vi "SP_OEE_2_test.vi"() -> ()   [LabVIEW 2017] (continued)
                      tunnel: w11433 -> [w11683]
                      tunnel: w11432 -> [w11682]
                      tunnel: w11431 -> [w11677]
                      tunnel: w11430 -> [w11679]
                      tunnel: w11429 -> [w11681]
                      tunnel: w11428 -> [w11680]
                      tunnel: w11427 -> [w11674]
                      tunnel: w11426 -> [w11675]
                      tunnel: [w11688] -> w11422
                      tunnel: [w11687] -> w11421
                      tunnel: [w11686] -> w11420
                      tunnel: [w11685] -> w11419
                      tunnel: [w11684] -> w11418
                      tunnel: [w11683] -> w11417
                      tunnel: [w11682] -> w11416
                      tunnel: [w11681] -> w11415
                      tunnel: [w11680] -> w11414
                      tunnel: [w11678] -> w11413
                      tunnel: [w11676] -> w11412
                      tunnel: [w11672] -> w11411
                      tunnel: [w11670] -> w11410
                      tunnel: w11425 -> [w11671]
                      tunnel: w11424 -> [w11667]
                      tunnel: [w11666] -> w11409
                      tunnel: w11423 -> [w11666]
                      tunnel: w11422 -> [w11727]
                      tunnel: w11421 -> [w11720]
                      tunnel: w11420 -> [w11711]
                      tunnel: w11419 -> [w11719]
                      tunnel: w11418 -> [w11709]
                      tunnel: w11417 -> [w11718]
                      tunnel: w11416 -> [w11707]
                      tunnel: w11415 -> [w11717]
                      tunnel: w11414 -> [w11705]
                      tunnel: w11413 -> [w11741]
                      tunnel: w11412 -> [w11740]
                      tunnel: w11411 -> [w11716]
                      tunnel: w11410 -> [w11703]
                      tunnel: [w11741] -> w11408
                      tunnel: [w11740] -> w11407
                      tunnel: [w11734] -> w11406
                      tunnel: [w11727] -> w11405
                      tunnel: [w11726] -> w11404
                      tunnel: [w11725] -> w11403
                      tunnel: [w11724] -> w11402
                      tunnel: [w11723] -> w11401
                      tunnel: [w11722] -> w11400
                      tunnel: [w11721] -> w11399
                      tunnel: [w11720] -> w11398
                      tunnel: [w11719] -> w11397
                      tunnel: [w11718] -> w11396
                      tunnel: [w11717] -> w11395
                      tunnel: [w11716] -> w11394
                      tunnel: [w11701] -> w11393
                      tunnel: w11409 -> [w11701]
                      tunnel: [w11754] -> _
                      tunnel: [w11748] -> _
                      tunnel: w11408 -> [w11749]
                      tunnel: w11407 -> [w11754]
                      tunnel: w11406 -> [w11743]
                      tunnel: w11405 -> [w11752]
                      tunnel: w11404 -> [w11750]
                      tunnel: w11403 -> [_]
                      tunnel: w11402 -> [_]
                      tunnel: w11401 -> [_]
                      tunnel: w11400 -> [_]
                      tunnel: w11399 -> [w11744]
                      tunnel: w11398 -> [w11751]
                      tunnel: w11397 -> [_]
                      tunnel: w11396 -> [_]
                      tunnel: w11395 -> [_]
                      tunnel: w11394 -> [_]
                      tunnel: w11393 -> [w11747]
                      frame #0 {
                        w11497 = "%Y-%m-%d" ("time format string (%c)")
                        n2093 = Decimal String To Number(string=w11483) -> (number=w11484:i32)  [unwired: 2 in, 1 out]
                        n2094 = property on="Table" class="Tbl (strict)"("Visible"=TRUE) -> ()  [unwired: 2 in, 2 out]
                        n2095 = Format Date/Time String(time format string (%c)=w11497, seconds (now)=w11489) -> (date/time string=w11498:string)  [unwired: 1 in]
                        n2096 = Format Date/Time String(time format string (%c)=w11497, seconds (now)=w11488) -> (date/time string=w11496:string)  [unwired: 1 in]
                        n2097 = Format Into String(format string="Where BREAKDOWN_DATE between '%s' and '%s' and  SHIFT_ID = '%d'  ", w11498, w11496, w11484) -> (resulting string=w11495:string)  [unwired: 2 in, 1 out]
                        n2098 = call <vilib>:"DB Tools Select Data.vi"("condition"=w11495, "error in (no error)"=w11504, "columns"=string[] ["BREAKDOWN_DATE"], "table"="STATION_1_LOG_HISTORY", "connection reference"=w11506) -> ("error out"=w11491:errorcluster, "data"=w11494:variant[][], "connection reference out"=w11505:T2)  [unwired: 1 in]
                        n2099 = property on="Table 2" class="Tbl (strict)"("Visible"=FALSE) -> ()  [unwired: 2 in, 2 out]
                        n2100 = xnode "Database Variant To Data"("database variant"=w11494, "error in (no error)"=w11491, "type"=string[][] [] ("Elements Found")) -> ("data"=w11492:string[][], "error out"=w11490:errorcluster)
                        n2101 = Index Array(array=w11492, index (col)=0 ("disabled index (col)")) -> (element=w11500:string[])  [unwired: 1 in]
                        n2102 = call "Search_1d_array_element.vi"("Count in"=string[] [] ("Elements Found"), "BD Date"=w11500, "Elements Found in"=string[] [] ("Elements Found")) -> ("Elements Found out"=w11487:string[])  [unwired: 4 in, 2 out]
                        n2103 = Build Array(w11487) -> (w11510:string[][])
                        n2104 = Transpose 2D Array(2D array=w11510) -> (transposed array=w11509:string[][])
                      }
                      frame #1 {
                        n2105 = call "Stack_holderwise_total_bd_count_&_duration_2.vi"("Refnum in"=w11572, "BREAKDOWN_STK_HOLD_ID"=1, "condition"=w11559, "Form Date"=w11566, "To Date"=w11565, "error in (no error)"=w11570, "Shift"=w11556) -> ("Refnum out"=w11571:T2, "Count out"=w11564:string[], "appended array"=w11561:dbl[], "error out"=w11569:errorcluster)  [unwired: 5 in]
                        n2106 = call "NUMERIC TO STRING.vi"("appended array"=w11561) -> ("Array"=w11560:string[])  [unwired: 4 in]
                        n2107 = call "Insert_empty_element_with_zero.vi"("searched date"=w11564, "fixed date"=w11562) -> ("O/P"=w11557:string[])  [unwired: 9 in]
                        n2108 = call "Insert_empty_element_with_zero.vi"("searched date"=w11560, "fixed date"=w11562) -> ("O/P"=w11563:string[])  [unwired: 9 in]
                      }
                      frame #2 {
                        n2109 = disable-structure shown="Enabled" {
                          disable-tunnel: w11586 -> [w11599 w11601]
                          disable-tunnel: [w11598 w11601] -> w11585
                          disable-tunnel: w11584 -> [w11597 w11600]
                          disable-tunnel: [w11595 w11600] -> w11583
                          disable-tunnel: w11582 -> [w11594 _]
                          disable-tunnel: w11581 -> [w11593 _]
                          disable-tunnel: [w11592 _] -> w11580
                          disable-tunnel: [w11591 _] -> w11576
                          disable-tunnel: w11574 -> [w11590 _]
                          frame Disabled {
                            n2110 = call "Stack_holderwise_total_bd_count_&_duration.vi"("Refnum in"=w11597, "BREAKDOWN_STK_HOLD_ID"=2, "condition"=w11590, "Form Date"=w11594, "To Date"=w11593, "error in (no error)"=w11599) -> ("Refnum out"=w11595:T2, "Count out"=w11592:string[], "appended array"=w11591:dbl[], "error out"=w11598:errorcluster)  [unwired: 6 in]
                          }
                          frame Enabled {
                          }
                        }
                        n2111 = call "Insert_empty_element_with_zero.vi"("searched date"=w11580, "fixed date"=w11577) -> ("O/P"=w11579:string[])  [unwired: 9 in]
                        n2112 = call "NUMERIC TO STRING.vi"("appended array"=w11576) -> ("Array"=w11575:string[])  [unwired: 4 in]
                        n2113 = call "Insert_empty_element_with_zero.vi"("searched date"=w11575, "fixed date"=w11577) -> ("O/P"=w11578:string[])  [unwired: 9 in]
                      }
                      frame #3 {
                        n2114 = disable-structure shown="Enabled" {
                          disable-tunnel: w11615 -> [w11629 w11632]
                          disable-tunnel: [w11628 w11632] -> w11614
                          disable-tunnel: w11613 -> [w11627 w11631]
                          disable-tunnel: [w11626 w11631] -> w11612
                          disable-tunnel: w11611 -> [w11625 _]
                          disable-tunnel: w11610 -> [w11624 _]
                          disable-tunnel: [w11623 _] -> w11609
                          disable-tunnel: [w11622 _] -> w11605
                          disable-tunnel: w11603 -> [w11621 _]
                          frame Disabled {
                            n2115 = call "Stack_holderwise_total_bd_count_&_duration.vi"("Refnum in"=w11627, "BREAKDOWN_STK_HOLD_ID"=3, "condition"=w11621, "Form Date"=w11625, "To Date"=w11624, "error in (no error)"=w11629) -> ("Refnum out"=w11626:T2, "Count out"=w11623:string[], "appended array"=w11622:dbl[], "error out"=w11628:errorcluster)  [unwired: 6 in]
                          }
                          frame Enabled {
                          }
                        }
                        n2116 = call "Insert_empty_element_with_zero.vi"("searched date"=w11609, "fixed date"=w11606) -> ("O/P"=w11608:string[])  [unwired: 9 in]
                        n2117 = call "NUMERIC TO STRING.vi"("appended array"=w11605) -> ("Array"=w11604:string[])  [unwired: 4 in]
                        n2118 = call "Insert_empty_element_with_zero.vi"("searched date"=w11604, "fixed date"=w11606) -> ("O/P"=w11607:string[])  [unwired: 9 in]
                      }
                      frame #4 {
                        n2119 = disable-structure shown="Enabled" {
                          disable-tunnel: w11646 -> [w11662 w11665]
                          disable-tunnel: w11645 -> [w11661 w11664]
                          disable-tunnel: [w11660 w11664] -> w11644
                          disable-tunnel: [w11659 w11665] -> w11643
                          disable-tunnel: w11642 -> [w11658 _]
                          disable-tunnel: w11641 -> [w11657 _]
                          disable-tunnel: [w11656 _] -> w11640
                          disable-tunnel: [w11655 _] -> w11636
                          disable-tunnel: w11634 -> [w11654 _]
                          frame Disabled {
                            n2120 = call "Stack_holderwise_total_bd_count_&_duration.vi"("Refnum in"=w11661, "BREAKDOWN_STK_HOLD_ID"=4, "condition"=w11654, "Form Date"=w11658, "To Date"=w11657, "error in (no error)"=w11662) -> ("Refnum out"=w11660:T2, "Count out"=w11656:string[], "appended array"=w11655:dbl[], "error out"=w11659:errorcluster)  [unwired: 6 in]
                          }
                          frame Enabled {
                          }
                        }
                        n2121 = call "Insert_empty_element_with_zero.vi"("searched date"=w11640, "fixed date"=w11637) -> ("O/P"=w11639:string[])  [unwired: 9 in]
                        n2122 = call "NUMERIC TO STRING.vi"("appended array"=w11636) -> ("Array"=w11635:string[])  [unwired: 4 in]
                        n2123 = call "Insert_empty_element_with_zero.vi"("searched date"=w11635, "fixed date"=w11637) -> ("O/P"=w11638:string[])  [unwired: 9 in]
                      }
                      frame #5 {
                        n2124 = disable-structure shown="Enabled" {
                          disable-tunnel: w11679 -> [w11697 w11700]
                          disable-tunnel: [w11696 w11700] -> w11678
                          disable-tunnel: w11677 -> [w11695 w11699]
                          disable-tunnel: [w11694 w11699] -> w11676
                          disable-tunnel: w11675 -> [w11693 _]
                          disable-tunnel: w11674 -> [w11692 _]
                          disable-tunnel: [w11691 _] -> w11673
                          disable-tunnel: [w11690 _] -> w11669
                          disable-tunnel: w11667 -> [w11689 _]
                          frame Disabled {
                            n2125 = call "Stack_holderwise_total_bd_count_&_duration.vi"("Refnum in"=w11695, "BREAKDOWN_STK_HOLD_ID"=5, "condition"=w11689, "Form Date"=w11692, "To Date"=w11693, "error in (no error)"=w11697) -> ("Refnum out"=w11694:T2, "Count out"=w11691:string[], "appended array"=w11690:dbl[], "error out"=w11696:errorcluster)  [unwired: 6 in]
                          }
                          frame Enabled {
                          }
                        }
                        n2126 = call "NUMERIC TO STRING.vi"("appended array"=w11669) -> ("Array"=w11668:string[])  [unwired: 4 in]
                        n2127 = call "Insert_empty_element_with_zero.vi"("searched date"=w11673, "fixed date"=w11671) -> ("O/P"=w11672:string[])  [unwired: 9 in]
                        n2128 = call "Insert_empty_element_with_zero.vi"("searched date"=w11668, "fixed date"=w11671) -> ("O/P"=w11670:string[])  [unwired: 9 in]
                      }
                      frame #6 {
                        n2129 = call "String to numeric.vi"("Array"=w11711) -> ("Array 2"=w11710:dbl[])  [unwired: 4 in]
                        n2130 = call "String to numeric.vi"("Array"=w11709) -> ("Array 2"=w11708:dbl[])  [unwired: 4 in]
                        n2131 = call "String to numeric.vi"("Array"=w11707) -> ("Array 2"=w11706:dbl[])  [unwired: 4 in]
                        n2132 = call "String to numeric.vi"("Array"=w11705) -> ("Array 2"=w11704:dbl[])  [unwired: 4 in]
                        n2133 = call "String to numeric.vi"("Array"=w11703) -> ("Array 2"=w11702:dbl[])  [unwired: 4 in]
                        n2134 = Decimal String To Number(string=w11716) -> (number=w11735:i32[])  [unwired: 2 in, 1 out]
                        n2135 = Decimal String To Number(string=w11717) -> (number=w11736:i32[])  [unwired: 2 in, 1 out]
                        n2136 = Decimal String To Number(string=w11718) -> (number=w11737:i32[])  [unwired: 2 in, 1 out]
                        n2137 = Decimal String To Number(string=w11719) -> (number=w11738:i32[])  [unwired: 2 in, 1 out]
                        n2138 = Decimal String To Number(string=w11720) -> (number=w11733:i32[])  [unwired: 2 in, 1 out]
                        n2139 = Compound Arithmetic op=ADD(w11710, w11708, w11706, w11704, w11702) -> (w11713:dbl[])
                        n2140 = Build Array(w11711) -> (w11732:string[][])
                        n2141 = Build Array(w11709) -> (w11731:string[][])
                        n2142 = Build Array(w11707) -> (w11730:string[][])
                        n2143 = Build Array(w11705) -> (w11729:string[][])
                        n2144 = Build Array(w11703) -> (w11728:string[][])
                        n2145 = Number To Fractional String(number=w11713, precision (6)=i16 2) -> (F-format string=w11712:string[])  [unwired: 2 in]
                        n2146 = Compound Arithmetic op=ADD(w11735, w11736, w11737, w11738, w11733) -> (w11739:i32[])
                        n2147 = Transpose 2D Array(2D array=w11732) -> (transposed array=w11726:string[][])
                        n2148 = Transpose 2D Array(2D array=w11731) -> (transposed array=w11725:string[][])
                        n2149 = Transpose 2D Array(2D array=w11730) -> (transposed array=w11724:string[][])
                        n2150 = Transpose 2D Array(2D array=w11729) -> (transposed array=w11723:string[][])
                        n2151 = Transpose 2D Array(2D array=w11728) -> (transposed array=w11722:string[][])
                        n2152 = Number To Decimal String(number=w11739) -> (decimal integer string=w11734:string[])  [unwired: 1 in]
                        n2153 = Build Array(w11712) -> (w11715:string[][])
                        n2154 = Transpose 2D Array(2D array=w11715) -> (transposed array=w11721:string[][])
                      }
                      frame #7 {
                        w11742 = string[] [""]
                        n2155 = Insert Into Array(array=w11752, index (col)=1 ("disabled index (col)"), new element #1=w11751, new element #2=w11750, new element #3=w11742, new element #4=w11742, new element #5=w11742, new element #6=w11742, new element #7=w11742, new element #8=w11742, new element #9=w11742, new element #10=w11742, new element #11=w11743, new element #12=w11744) -> (w11746:string[][])  [unwired: 1 in]
                        n2156 = call "flot graph for month n year.vi"("BD Date"=w11747, "error in (no error)"=w11749, "Count total"=w11743) -> ("error out"=w11748:errorcluster, "Run-Time Status"=w11745:cluster{"Array 2":timestamp[], dbl[]})  [unwired: 7 in]
                        n2157 = local write "Run-Time Status"(w11745) -> ()
                        n2158 = local write "Table"(w11746) -> ()
                      }
                    }
                  }
                  frame "3" {
                    n2159 = flat-sequence {
                      tunnel: w11761 -> [w11875]
                      tunnel: w11760 -> [w11873]
                      tunnel: [w11859] -> w11851
                      tunnel: [w11874] -> w11850
                      tunnel: w11759 -> [_]
                      tunnel: [w11878] -> w11849
                      tunnel: [w11858] -> w11848
                      tunnel: [w11857] -> w11847
                      tunnel: [w11856] -> w11846
                      tunnel: w11758 -> [w11858]
                      tunnel: w11757 -> [w11857]
                      tunnel: ["Where BREAKDOWN_DATE between '%s'and '%s' and BREAKDOWN_STK_HOLD_ID ='%d' and  SHIFT_ID = '%d' "] -> w11845
                      tunnel: [w11856] -> w11844
                      tunnel: w11756 -> [w11852]
                      tunnel: [w11852] -> w11755
                      tunnel: w11851 -> [w11939]
                      tunnel: w11850 -> [w11941]
                      tunnel: w11849 -> [w11936]
                      tunnel: w11848 -> [w11935]
                      tunnel: w11847 -> [w11934]
                      tunnel: [w11938] -> w11843
                      tunnel: [w11940] -> w11842
                      tunnel: [w11936] -> w11841
                      tunnel: [w11926] -> w11840
                      tunnel: [w11932] -> w11839
                      tunnel: [w11935] -> w11838
                      tunnel: [w11934] -> w11837
                      tunnel: w11846 -> [w11931]
                      tunnel: [w11931] -> w11836
                      tunnel: w11845 -> [w11928]
                      tunnel: [w11928] -> w11835
                      tunnel: [w11927] -> w11834
                      tunnel: w11844 -> [w11927]
                      tunnel: w11755 -> [w11925]
                      tunnel: w11843 -> [w11955]
                      tunnel: w11842 -> [w11953]
                      tunnel: w11841 -> [w11958]
                      tunnel: w11840 -> [w11957]
                      tunnel: w11839 -> [w11956]
                      tunnel: w11838 -> [w11951]
                      tunnel: w11837 -> [w11950]
                      tunnel: [w11958] -> w11833
                      tunnel: [w11957] -> w11832
                      tunnel: [w11956] -> w11831
                      tunnel: [w11954] -> w11830
                      tunnel: [w11948] -> w11829
                      tunnel: [w11947] -> w11828
                      tunnel: [w11952] -> w11827
                      tunnel: [w11951] -> w11826
                      tunnel: [w11950] -> w11825
                      tunnel: w11836 -> [w11946]
                      tunnel: [w11946] -> w11824
                      tunnel: w11835 -> [w11943]
                      tunnel: [w11943] -> w11823
                      tunnel: [w11942] -> w11822
                      tunnel: w11834 -> [w11942]
                      tunnel: w11833 -> [w11989]
                      tunnel: w11832 -> [w11988]
                      tunnel: w11831 -> [w11987]
                      tunnel: w11830 -> [w11984]
                      tunnel: w11829 -> [w11986]
                      tunnel: w11828 -> [w11985]
                      tunnel: w11827 -> [w11982]
                      tunnel: w11826 -> [w11980]
                      tunnel: w11825 -> [w11979]
                      tunnel: [w11989] -> w11821
                      tunnel: [w11988] -> w11820
                      tunnel: [w11987] -> w11819
                      tunnel: [w11986] -> w11818
                      tunnel: [w11985] -> w11817
                      tunnel: [w11983] -> w11816
                      tunnel: [w11977] -> w11815
                      tunnel: [w11976] -> w11814
                      tunnel: [w11981] -> w11813
                      tunnel: [w11980] -> w11812
                      tunnel: [w11979] -> w11811
                      tunnel: w11824 -> [w11975]
                      tunnel: [w11975] -> w11810
                      tunnel: w11823 -> [w11972]
                      tunnel: [w11972] -> w11809
                      tunnel: [w11971] -> w11808
                      tunnel: w11822 -> [w11971]
                      tunnel: w11821 -> [w12022]
                      tunnel: w11820 -> [w12021]
                      tunnel: w11819 -> [w12020]
                      tunnel: w11818 -> [w12019]
                      tunnel: w11817 -> [w12018]
                      tunnel: w11816 -> [w12015]
                      tunnel: w11815 -> [w12017]
                      tunnel: w11814 -> [w12016]
                      tunnel: w11813 -> [w12014]
                      tunnel: w11812 -> [w12011]
                      tunnel: w11811 -> [w12010]
                      tunnel: [w12022] -> w11807
                      tunnel: [w12021] -> w11806
                      tunnel: [w12020] -> w11805
                      tunnel: [w12019] -> w11804
                      tunnel: [w12018] -> w11803
                      tunnel: [w12017] -> w11802
                      tunnel: [w12016] -> w11801
                      tunnel: [w12013] -> w11800
                      tunnel: [w12012] -> w11799
                      tunnel: [w12008] -> w11798
                      tunnel: [w12007] -> w11797
                      tunnel: [w12011] -> w11796
                      tunnel: [w12010] -> w11795
                      tunnel: w11810 -> [w12006]
                      tunnel: [w12006] -> w11794
                      tunnel: w11809 -> [w12003]
                      tunnel: [w12003] -> w11793
                      tunnel: [w12002] -> w11792
                      tunnel: w11808 -> [w12002]
                      tunnel: w11807 -> [w12057]
                      tunnel: w11806 -> [w12056]
                      tunnel: w11805 -> [w12055]
                      tunnel: w11804 -> [w12054]
                      tunnel: w11803 -> [w12053]
                      tunnel: w11802 -> [w12052]
                      tunnel: w11801 -> [w12051]
                      tunnel: w11800 -> [w12046]
                      tunnel: w11799 -> [w12048]
                      tunnel: w11798 -> [w12050]
                      tunnel: w11797 -> [w12049]
                      tunnel: w11796 -> [w12043]
                      tunnel: w11795 -> [w12044]
                      tunnel: [w12057] -> w11791
                      tunnel: [w12056] -> w11790
                      tunnel: [w12055] -> w11789
                      tunnel: [w12054] -> w11788
                      tunnel: [w12053] -> w11787
                      tunnel: [w12052] -> w11786
                      tunnel: [w12051] -> w11785
                      tunnel: [w12050] -> w11784
                      tunnel: [w12049] -> w11783
                      tunnel: [w12047] -> w11782
                      tunnel: [w12045] -> w11781
                      tunnel: [w12041] -> w11780
                      tunnel: [w12039] -> w11779
                      tunnel: w11794 -> [w12040]
                      tunnel: w11793 -> [w12036]
                      tunnel: [w12035] -> w11778
                      tunnel: w11792 -> [w12035]
                      tunnel: w11791 -> [w12096]
                      tunnel: w11790 -> [w12089]
                      tunnel: w11789 -> [w12080]
                      tunnel: w11788 -> [w12088]
                      tunnel: w11787 -> [w12078]
                      tunnel: w11786 -> [w12087]
                      tunnel: w11785 -> [w12076]
                      tunnel: w11784 -> [w12086]
                      tunnel: w11783 -> [w12074]
                      tunnel: w11782 -> [w12110]
                      tunnel: w11781 -> [w12109]
                      tunnel: w11780 -> [w12085]
                      tunnel: w11779 -> [w12072]
                      tunnel: [w12110] -> w11777
                      tunnel: [w12109] -> w11776
                      tunnel: [w12103] -> w11775
                      tunnel: [w12096] -> w11774
                      tunnel: [w12095] -> w11773
                      tunnel: [w12094] -> w11772
                      tunnel: [w12093] -> w11771
                      tunnel: [w12092] -> w11770
                      tunnel: [w12091] -> w11769
                      tunnel: [w12090] -> w11768
                      tunnel: [w12089] -> w11767
                      tunnel: [w12088] -> w11766
                      tunnel: [w12087] -> w11765
                      tunnel: [w12086] -> w11764
                      tunnel: [w12085] -> w11763
                      tunnel: [w12070] -> w11762
                      tunnel: w11778 -> [w12070]
                      tunnel: [w12123] -> _
                      tunnel: [w12117] -> _
                      tunnel: w11777 -> [w12118]
                      tunnel: w11776 -> [w12123]
                      tunnel: w11775 -> [w12112]
                      tunnel: w11774 -> [w12121]
                      tunnel: w11773 -> [w12119]
                      tunnel: w11772 -> [_]
                      tunnel: w11771 -> [_]
                      tunnel: w11770 -> [_]
                      tunnel: w11769 -> [_]
                      tunnel: w11768 -> [w12113]
                      tunnel: w11767 -> [w12120]
                      tunnel: w11766 -> [_]
                      tunnel: w11765 -> [_]
                      tunnel: w11764 -> [_]
                      tunnel: w11763 -> [_]
                      tunnel: w11762 -> [w12116]
                      frame #0 {
                        w11866 = "%Y-%m-%d" ("time format string (%c)")
                        n2160 = Decimal String To Number(string=w11852) -> (number=w11853:i32)  [unwired: 2 in, 1 out]
                        n2161 = property on="Table" class="Tbl (strict)"("Visible"=TRUE) -> ()  [unwired: 2 in, 2 out]
                        n2162 = Format Date/Time String(time format string (%c)=w11866, seconds (now)=w11858) -> (date/time string=w11867:string)  [unwired: 1 in]
                        n2163 = Format Date/Time String(time format string (%c)=w11866, seconds (now)=w11857) -> (date/time string=w11865:string)  [unwired: 1 in]
                        n2164 = Format Into String(format string="Where BREAKDOWN_DATE between '%s' and '%s' and  SHIFT_ID = '%d'  ", w11867, w11865, w11853) -> (resulting string=w11864:string)  [unwired: 2 in, 1 out]
                        n2165 = call <vilib>:"DB Tools Select Data.vi"("condition"=w11864, "error in (no error)"=w11873, "columns"=string[] ["BREAKDOWN_DATE"], "table"="STATION_1_LOG_HISTORY", "connection reference"=w11875) -> ("error out"=w11860:errorcluster, "data"=w11863:variant[][], "connection reference out"=w11874:T2)  [unwired: 1 in]
                        n2166 = property on="Table 2" class="Tbl (strict)"("Visible"=FALSE) -> ()  [unwired: 2 in, 2 out]
                        n2167 = xnode "Database Variant To Data"("database variant"=w11863, "error in (no error)"=w11860, "type"=string[][] [] ("Elements Found")) -> ("data"=w11861:string[][], "error out"=w11859:errorcluster)
                        n2168 = Index Array(array=w11861, index (col)=0 ("disabled index (col)")) -> (element=w11869:string[])  [unwired: 1 in]
                        n2169 = call "Search_1d_array_element.vi"("Count in"=string[] [] ("Elements Found"), "BD Date"=w11869, "Elements Found in"=string[] [] ("Elements Found")) -> ("Elements Found out"=w11856:string[])  [unwired: 4 in, 2 out]
                        n2170 = Build Array(w11856) -> (w11879:string[][])
                        n2171 = Transpose 2D Array(2D array=w11879) -> (transposed array=w11878:string[][])
                      }
                      frame #1 {
                        n2172 = call "Stack_holderwise_total_bd_count_&_duration_2.vi"("Refnum in"=w11941, "BREAKDOWN_STK_HOLD_ID"=1, "condition"=w11928, "Form Date"=w11935, "To Date"=w11934, "error in (no error)"=w11939, "Shift"=w11925) -> ("Refnum out"=w11940:T2, "Count out"=w11933:string[], "appended array"=w11930:dbl[], "error out"=w11938:errorcluster)  [unwired: 5 in]
                        n2173 = call "NUMERIC TO STRING.vi"("appended array"=w11930) -> ("Array"=w11929:string[])  [unwired: 4 in]
                        n2174 = call "Insert_empty_element_with_zero.vi"("searched date"=w11933, "fixed date"=w11931) -> ("O/P"=w11926:string[])  [unwired: 9 in]
                        n2175 = call "Insert_empty_element_with_zero.vi"("searched date"=w11929, "fixed date"=w11931) -> ("O/P"=w11932:string[])  [unwired: 9 in]
                      }
                      frame #2 {
                        n2176 = disable-structure shown="Enabled" {
                          disable-tunnel: w11955 -> [w11968 w11970]
                          disable-tunnel: [w11967 w11970] -> w11954
                          disable-tunnel: w11953 -> [w11966 w11969]
                          disable-tunnel: [w11964 w11969] -> w11952
                          disable-tunnel: w11951 -> [w11963 _]
                          disable-tunnel: w11950 -> [w11962 _]
                          disable-tunnel: [w11961 _] -> w11949
                          disable-tunnel: [w11960 _] -> w11945
                          disable-tunnel: w11943 -> [w11959 _]
                          frame Disabled {
                            n2177 = call "Stack_holderwise_total_bd_count_&_duration.vi"("Refnum in"=w11966, "BREAKDOWN_STK_HOLD_ID"=2, "condition"=w11959, "Form Date"=w11963, "To Date"=w11962, "error in (no error)"=w11968) -> ("Refnum out"=w11964:T2, "Count out"=w11961:string[], "appended array"=w11960:dbl[], "error out"=w11967:errorcluster)  [unwired: 6 in]
                          }
                          frame Enabled {
                          }
                        }
                        n2178 = call "Insert_empty_element_with_zero.vi"("searched date"=w11949, "fixed date"=w11946) -> ("O/P"=w11948:string[])  [unwired: 9 in]
                        n2179 = call "NUMERIC TO STRING.vi"("appended array"=w11945) -> ("Array"=w11944:string[])  [unwired: 4 in]
                        n2180 = call "Insert_empty_element_with_zero.vi"("searched date"=w11944, "fixed date"=w11946) -> ("O/P"=w11947:string[])  [unwired: 9 in]
                      }
                      frame #3 {
                        n2181 = disable-structure shown="Enabled" {
                          disable-tunnel: w11984 -> [w11998 w12001]
                          disable-tunnel: [w11997 w12001] -> w11983
                          disable-tunnel: w11982 -> [w11996 w12000]
                          disable-tunnel: [w11995 w12000] -> w11981
                          disable-tunnel: w11980 -> [w11994 _]
                          disable-tunnel: w11979 -> [w11993 _]
                          disable-tunnel: [w11992 _] -> w11978
                          disable-tunnel: [w11991 _] -> w11974
                          disable-tunnel: w11972 -> [w11990 _]
                          frame Disabled {
                            n2182 = call "Stack_holderwise_total_bd_count_&_duration.vi"("Refnum in"=w11996, "BREAKDOWN_STK_HOLD_ID"=3, "condition"=w11990, "Form Date"=w11994, "To Date"=w11993, "error in (no error)"=w11998) -> ("Refnum out"=w11995:T2, "Count out"=w11992:string[], "appended array"=w11991:dbl[], "error out"=w11997:errorcluster)  [unwired: 6 in]
                          }
                          frame Enabled {
                          }
                        }
                        n2183 = call "Insert_empty_element_with_zero.vi"("searched date"=w11978, "fixed date"=w11975) -> ("O/P"=w11977:string[])  [unwired: 9 in]
                        n2184 = call "NUMERIC TO STRING.vi"("appended array"=w11974) -> ("Array"=w11973:string[])  [unwired: 4 in]
                        n2185 = call "Insert_empty_element_with_zero.vi"("searched date"=w11973, "fixed date"=w11975) -> ("O/P"=w11976:string[])  [unwired: 9 in]
                      }
                      frame #4 {
                        n2186 = disable-structure shown="Enabled" {
                          disable-tunnel: w12015 -> [w12031 w12034]
                          disable-tunnel: w12014 -> [w12030 w12033]
                          disable-tunnel: [w12029 w12033] -> w12013
                          disable-tunnel: [w12028 w12034] -> w12012
                          disable-tunnel: w12011 -> [w12027 _]
                          disable-tunnel: w12010 -> [w12026 _]
                          disable-tunnel: [w12025 _] -> w12009
                          disable-tunnel: [w12024 _] -> w12005
                          disable-tunnel: w12003 -> [w12023 _]
                          frame Disabled {
                            n2187 = call "Stack_holderwise_total_bd_count_&_duration.vi"("Refnum in"=w12030, "BREAKDOWN_STK_HOLD_ID"=4, "condition"=w12023, "Form Date"=w12027, "To Date"=w12026, "error in (no error)"=w12031) -> ("Refnum out"=w12029:T2, "Count out"=w12025:string[], "appended array"=w12024:dbl[], "error out"=w12028:errorcluster)  [unwired: 6 in]
                          }
                          frame Enabled {
                          }
                        }
                        n2188 = call "Insert_empty_element_with_zero.vi"("searched date"=w12009, "fixed date"=w12006) -> ("O/P"=w12008:string[])  [unwired: 9 in]
                        n2189 = call "NUMERIC TO STRING.vi"("appended array"=w12005) -> ("Array"=w12004:string[])  [unwired: 4 in]
                        n2190 = call "Insert_empty_element_with_zero.vi"("searched date"=w12004, "fixed date"=w12006) -> ("O/P"=w12007:string[])  [unwired: 9 in]
                      }
                      frame #5 {
                        n2191 = disable-structure shown="Enabled" {
                          disable-tunnel: w12048 -> [w12066 w12069]
                          disable-tunnel: [w12065 w12069] -> w12047
                          disable-tunnel: w12046 -> [w12064 w12068]
                          disable-tunnel: [w12063 w12068] -> w12045
                          disable-tunnel: w12044 -> [w12062 _]
                          disable-tunnel: w12043 -> [w12061 _]
                          disable-tunnel: [w12060 _] -> w12042
                          disable-tunnel: [w12059 _] -> w12038
                          disable-tunnel: w12036 -> [w12058 _]
                          frame Disabled {
                            n2192 = call "Stack_holderwise_total_bd_count_&_duration.vi"("Refnum in"=w12064, "BREAKDOWN_STK_HOLD_ID"=5, "condition"=w12058, "Form Date"=w12061, "To Date"=w12062, "error in (no error)"=w12066) -> ("Refnum out"=w12063:T2, "Count out"=w12060:string[], "appended array"=w12059:dbl[], "error out"=w12065:errorcluster)  [unwired: 6 in]
                          }
                          frame Enabled {
                          }
                        }
                        n2193 = call "NUMERIC TO STRING.vi"("appended array"=w12038) -> ("Array"=w12037:string[])  [unwired: 4 in]
                        n2194 = call "Insert_empty_element_with_zero.vi"("searched date"=w12042, "fixed date"=w12040) -> ("O/P"=w12041:string[])  [unwired: 9 in]
                        n2195 = call "Insert_empty_element_with_zero.vi"("searched date"=w12037, "fixed date"=w12040) -> ("O/P"=w12039:string[])  [unwired: 9 in]
                      }
                      frame #6 {
                        n2196 = call "String to numeric.vi"("Array"=w12080) -> ("Array 2"=w12079:dbl[])  [unwired: 4 in]
                        n2197 = call "String to numeric.vi"("Array"=w12078) -> ("Array 2"=w12077:dbl[])  [unwired: 4 in]
                        n2198 = call "String to numeric.vi"("Array"=w12076) -> ("Array 2"=w12075:dbl[])  [unwired: 4 in]
                        n2199 = call "String to numeric.vi"("Array"=w12074) -> ("Array 2"=w12073:dbl[])  [unwired: 4 in]
                        n2200 = call "String to numeric.vi"("Array"=w12072) -> ("Array 2"=w12071:dbl[])  [unwired: 4 in]
                        n2201 = Decimal String To Number(string=w12085) -> (number=w12104:i32[])  [unwired: 2 in, 1 out]
                        n2202 = Decimal String To Number(string=w12086) -> (number=w12105:i32[])  [unwired: 2 in, 1 out]
                        n2203 = Decimal String To Number(string=w12087) -> (number=w12106:i32[])  [unwired: 2 in, 1 out]
                        n2204 = Decimal String To Number(string=w12088) -> (number=w12107:i32[])  [unwired: 2 in, 1 out]
                        n2205 = Decimal String To Number(string=w12089) -> (number=w12102:i32[])  [unwired: 2 in, 1 out]
                        n2206 = Compound Arithmetic op=ADD(w12079, w12077, w12075, w12073, w12071) -> (w12082:dbl[])
                        n2207 = Build Array(w12080) -> (w12101:string[][])
                        n2208 = Build Array(w12078) -> (w12100:string[][])
                        n2209 = Build Array(w12076) -> (w12099:string[][])
                        n2210 = Build Array(w12074) -> (w12098:string[][])
                        n2211 = Build Array(w12072) -> (w12097:string[][])
                        n2212 = Number To Fractional String(number=w12082, precision (6)=i16 2) -> (F-format string=w12081:string[])  [unwired: 2 in]
                        n2213 = Compound Arithmetic op=ADD(w12104, w12105, w12106, w12107, w12102) -> (w12108:i32[])
                        n2214 = Transpose 2D Array(2D array=w12101) -> (transposed array=w12095:string[][])
                        n2215 = Transpose 2D Array(2D array=w12100) -> (transposed array=w12094:string[][])
                        n2216 = Transpose 2D Array(2D array=w12099) -> (transposed array=w12093:string[][])
                        n2217 = Transpose 2D Array(2D array=w12098) -> (transposed array=w12092:string[][])
                        n2218 = Transpose 2D Array(2D array=w12097) -> (transposed array=w12091:string[][])
                        n2219 = Number To Decimal String(number=w12108) -> (decimal integer string=w12103:string[])  [unwired: 1 in]
                        n2220 = Build Array(w12081) -> (w12084:string[][])
                        n2221 = Transpose 2D Array(2D array=w12084) -> (transposed array=w12090:string[][])
                      }
                      frame #7 {
                        w12111 = string[] [""]
                        n2222 = Insert Into Array(array=w12121, index (col)=1 ("disabled index (col)"), new element #1=w12120, new element #2=w12119, new element #3=w12111, new element #4=w12111, new element #5=w12111, new element #6=w12111, new element #7=w12111, new element #8=w12111, new element #9=w12111, new element #10=w12111, new element #11=w12112, new element #12=w12113) -> (w12115:string[][])  [unwired: 1 in]
                        n2223 = call "flot graph for month n year.vi"("BD Date"=w12116, "error in (no error)"=w12118, "Count total"=w12112) -> ("error out"=w12117:errorcluster, "Run-Time Status"=w12114:cluster{"Array 2":timestamp[], dbl[]})  [unwired: 7 in]
                        n2224 = local write "Run-Time Status"(w12114) -> ()
                        n2225 = local write "Table"(w12115) -> ()
                      }
                    }
                  }
                  frame "all" {
                  }
                }
              }
              frame "Logistics" {
                n2226 = local read "Shift"() -> (w12126:string)
                n2227 = case shown="\"1\"" w12126 {
                  selector: w12126 -> [_ w12500 w12874 w13248 _]
                  tunnel: w12131 -> [w12136 w12505 w12879 w13253 _]
                  tunnel: w12130 -> [w12135 w12504 w12878 w13252 _]
                  tunnel: w12129 -> [w12134 w12503 w12877 w13251 _]
                  tunnel: w12128 -> [w12133 w12502 w12876 w13250 _]
                  tunnel: w12127 -> [w12132 w12501 w12875 w13249 _]
                  tunnel: [_ w12497 _ _ _] -> w12125
                  tunnel: [_ w12496 _ _ _] -> w12124
                  frame "ALL", Default {
                    n2228 = flat-sequence {
                      tunnel: w12136 -> [w12248]
                      tunnel: w12135 -> [w12246]
                      tunnel: [w12232] -> w12226
                      tunnel: [w12247] -> w12225
                      tunnel: w12134 -> [_]
                      tunnel: [w12251] -> w12224
                      tunnel: [w12231] -> w12223
                      tunnel: [w12230] -> w12222
                      tunnel: [w12228] -> w12221
                      tunnel: w12133 -> [w12231]
                      tunnel: w12132 -> [w12230]
                      tunnel: ["Where BREAKDOWN_DATE between '%s'and '%s' and BREAKDOWN_STK_HOLD_ID ='%d'  "] -> w12220
                      tunnel: [w12228] -> w12219
                      tunnel: w12226 -> [w12310]
                      tunnel: w12225 -> [w12312]
                      tunnel: w12224 -> [w12308]
                      tunnel: w12223 -> [w12307]
                      tunnel: w12222 -> [w12306]
                      tunnel: [w12309] -> w12218
                      tunnel: [w12311] -> w12217
                      tunnel: [w12308] -> w12216
                      tunnel: [w12298] -> w12215
                      tunnel: [w12304] -> w12214
                      tunnel: [w12307] -> w12213
                      tunnel: [w12306] -> w12212
                      tunnel: w12221 -> [w12303]
                      tunnel: [w12303] -> w12211
                      tunnel: w12220 -> [w12300]
                      tunnel: [w12300] -> w12210
                      tunnel: [w12299] -> w12209
                      tunnel: w12219 -> [w12299]
                      tunnel: w12218 -> [w12339]
                      tunnel: w12217 -> [w12337]
                      tunnel: w12216 -> [w12342]
                      tunnel: w12215 -> [w12341]
                      tunnel: w12214 -> [w12340]
                      tunnel: w12213 -> [w12335]
                      tunnel: w12212 -> [w12334]
                      tunnel: [w12342] -> w12208
                      tunnel: [w12341] -> w12207
                      tunnel: [w12340] -> w12206
                      tunnel: [w12338] -> w12205
                      tunnel: [w12332] -> w12204
                      tunnel: [w12331] -> w12203
                      tunnel: [w12336] -> w12202
                      tunnel: [w12335] -> w12201
                      tunnel: [w12334] -> w12200
                      tunnel: w12211 -> [w12330]
                      tunnel: [w12330] -> w12199
                      tunnel: w12210 -> [w12327]
                      tunnel: [w12327] -> w12198
                      tunnel: [w12326] -> w12197
                      tunnel: w12209 -> [w12326]
                      tunnel: w12208 -> [w12361]
                      tunnel: w12207 -> [w12360]
                      tunnel: w12206 -> [w12359]
                      tunnel: w12205 -> [w12356]
                      tunnel: w12204 -> [w12358]
                      tunnel: w12203 -> [w12357]
                      tunnel: w12202 -> [w12354]
                      tunnel: w12201 -> [w12352]
                      tunnel: w12200 -> [w12351]
                      tunnel: [w12361] -> w12196
                      tunnel: [w12360] -> w12195
                      tunnel: [w12359] -> w12194
                      tunnel: [w12358] -> w12193
                      tunnel: [w12357] -> w12192
                      tunnel: [w12355] -> w12191
                      tunnel: [w12349] -> w12190
                      tunnel: [w12348] -> w12189
                      tunnel: [w12353] -> w12188
                      tunnel: [w12352] -> w12187
                      tunnel: [w12351] -> w12186
                      tunnel: w12199 -> [w12347]
                      tunnel: [w12347] -> w12185
                      tunnel: w12198 -> [w12344]
                      tunnel: [w12344] -> w12184
                      tunnel: [w12343] -> w12183
                      tunnel: w12197 -> [w12343]
                      tunnel: w12196 -> [w12394]
                      tunnel: w12195 -> [w12393]
                      tunnel: w12194 -> [w12392]
                      tunnel: w12193 -> [w12391]
                      tunnel: w12192 -> [w12390]
                      tunnel: w12191 -> [w12387]
                      tunnel: w12190 -> [w12389]
                      tunnel: w12189 -> [w12388]
                      tunnel: w12188 -> [w12386]
                      tunnel: w12187 -> [w12383]
                      tunnel: w12186 -> [w12382]
                      tunnel: [w12394] -> w12182
                      tunnel: [w12393] -> w12181
                      tunnel: [w12392] -> w12180
                      tunnel: [w12391] -> w12179
                      tunnel: [w12390] -> w12178
                      tunnel: [w12389] -> w12177
                      tunnel: [w12388] -> w12176
                      tunnel: [w12385] -> w12175
                      tunnel: [w12384] -> w12174
                      tunnel: [w12380] -> w12173
                      tunnel: [w12379] -> w12172
                      tunnel: [w12383] -> w12171
                      tunnel: [w12382] -> w12170
                      tunnel: w12185 -> [w12378]
                      tunnel: [w12378] -> w12169
                      tunnel: w12184 -> [w12375]
                      tunnel: [w12375] -> w12168
                      tunnel: [w12374] -> w12167
                      tunnel: w12183 -> [w12374]
                      tunnel: w12182 -> [w12429]
                      tunnel: w12181 -> [w12428]
                      tunnel: w12180 -> [w12427]
                      tunnel: w12179 -> [w12426]
                      tunnel: w12178 -> [w12425]
                      tunnel: w12177 -> [w12424]
                      tunnel: w12176 -> [w12423]
                      tunnel: w12175 -> [w12418]
                      tunnel: w12174 -> [w12420]
                      tunnel: w12173 -> [w12422]
                      tunnel: w12172 -> [w12421]
                      tunnel: w12171 -> [w12415]
                      tunnel: w12170 -> [w12416]
                      tunnel: [w12429] -> w12166
                      tunnel: [w12428] -> w12165
                      tunnel: [w12427] -> w12164
                      tunnel: [w12426] -> w12163
                      tunnel: [w12425] -> w12162
                      tunnel: [w12424] -> w12161
                      tunnel: [w12423] -> w12160
                      tunnel: [w12422] -> w12159
                      tunnel: [w12421] -> w12158
                      tunnel: [w12419] -> w12157
                      tunnel: [w12417] -> w12156
                      tunnel: [w12413] -> w12155
                      tunnel: [w12411] -> w12154
                      tunnel: w12169 -> [w12412]
                      tunnel: w12168 -> [w12408]
                      tunnel: [w12407] -> w12153
                      tunnel: w12167 -> [w12407]
                      tunnel: w12166 -> [w12468]
                      tunnel: w12165 -> [w12461]
                      tunnel: w12164 -> [w12452]
                      tunnel: w12163 -> [w12460]
                      tunnel: w12162 -> [w12450]
                      tunnel: w12161 -> [w12459]
                      tunnel: w12160 -> [w12448]
                      tunnel: w12159 -> [w12458]
                      tunnel: w12158 -> [w12446]
                      tunnel: w12157 -> [w12482]
                      tunnel: w12156 -> [w12481]
                      tunnel: w12155 -> [w12457]
                      tunnel: w12154 -> [w12444]
                      tunnel: [w12482] -> w12152
                      tunnel: [w12481] -> w12151
                      tunnel: [w12475] -> w12150
                      tunnel: [w12468] -> w12149
                      tunnel: [w12467] -> w12148
                      tunnel: [w12466] -> w12147
                      tunnel: [w12465] -> w12146
                      tunnel: [w12464] -> w12145
                      tunnel: [w12463] -> w12144
                      tunnel: [w12462] -> w12143
                      tunnel: [w12461] -> w12142
                      tunnel: [w12460] -> w12141
                      tunnel: [w12459] -> w12140
                      tunnel: [w12458] -> w12139
                      tunnel: [w12457] -> w12138
                      tunnel: [w12442] -> w12137
                      tunnel: w12153 -> [w12442]
                      tunnel: [w12495] -> _
                      tunnel: [w12491] -> _
                      tunnel: w12152 -> [w12492]
                      tunnel: w12151 -> [w12495]
                      tunnel: w12150 -> [w12486]
                      tunnel: w12149 -> [w12493]
                      tunnel: w12148 -> [_]
                      tunnel: w12147 -> [w12484]
                      tunnel: w12146 -> [_]
                      tunnel: w12145 -> [_]
                      tunnel: w12144 -> [_]
                      tunnel: w12143 -> [w12487]
                      tunnel: w12142 -> [_]
                      tunnel: w12141 -> [w12485]
                      tunnel: w12140 -> [_]
                      tunnel: w12139 -> [_]
                      tunnel: w12138 -> [_]
                      tunnel: w12137 -> [w12490]
                      frame #0 {
                        w12239 = "%Y-%m-%d" ("time format string (%c)")
                        n2229 = property on="Table" class="Tbl (strict)"("Visible"=TRUE) -> ()  [unwired: 2 in, 2 out]
                        n2230 = Format Date/Time String(time format string (%c)=w12239, seconds (now)=w12231) -> (date/time string=w12240:string)  [unwired: 1 in]
                        n2231 = Format Date/Time String(time format string (%c)=w12239, seconds (now)=w12230) -> (date/time string=w12238:string)  [unwired: 1 in]
                        n2232 = Format Into String(format string="Where BREAKDOWN_DATE between '%s' and '%s' ", w12240, w12238) -> (resulting string=w12237:string)  [unwired: 2 in, 1 out]
                        n2233 = call <vilib>:"DB Tools Select Data.vi"("condition"=w12237, "error in (no error)"=w12246, "columns"=string[] ["BREAKDOWN_DATE"], "table"="STATION_1_LOG_HISTORY", "connection reference"=w12248) -> ("error out"=w12233:errorcluster, "data"=w12236:variant[][], "connection reference out"=w12247:T2)  [unwired: 1 in]
                        n2234 = property on="Table 2" class="Tbl (strict)"("Visible"=FALSE) -> ()  [unwired: 2 in, 2 out]
                        n2235 = xnode "Database Variant To Data"("database variant"=w12236, "error in (no error)"=w12233, "type"=string[][] [] ("Elements Found")) -> ("data"=w12234:string[][], "error out"=w12232:errorcluster)
                        n2236 = Index Array(array=w12234, index (col)=0 ("disabled index (col)")) -> (element=w12242:string[])  [unwired: 1 in]
                        n2237 = call "Search_1d_array_element.vi"("Count in"=string[] [] ("Elements Found"), "BD Date"=w12242, "Elements Found in"=string[] [] ("Elements Found")) -> ("Elements Found out"=w12228:string[])  [unwired: 4 in, 2 out]
                        n2238 = Build Array(w12228) -> (w12252:string[][])
                        n2239 = Transpose 2D Array(2D array=w12252) -> (transposed array=w12251:string[][])
                      }
                      frame #1 {
                        n2240 = disable-structure shown="Enabled" {
                          disable-tunnel: w12312 -> [w12322 w12323]
                          disable-tunnel: [w12321 w12323] -> w12311
                          disable-tunnel: w12310 -> [w12320 w12324]
                          disable-tunnel: [w12319 w12324] -> w12309
                          disable-tunnel: w12307 -> [w12317 _]
                          disable-tunnel: w12306 -> [w12316 _]
                          disable-tunnel: [w12315 _] -> w12305
                          disable-tunnel: [w12314 _] -> w12302
                          disable-tunnel: w12300 -> [w12313 _]
                          frame Disabled {
                            n2241 = call "Stack_holderwise_total_bd_count_&_duration.vi"("Refnum in"=w12322, "BREAKDOWN_STK_HOLD_ID"=1, "condition"=w12313, "Form Date"=w12317, "To Date"=w12316, "error in (no error)"=w12320) -> ("Refnum out"=w12321:T2, "Count out"=w12315:string[], "appended array"=w12314:dbl[], "error out"=w12319:errorcluster)  [unwired: 6 in]
                          }
                          frame Enabled {
                          }
                        }
                        n2242 = call "NUMERIC TO STRING.vi"("appended array"=w12302) -> ("Array"=w12301:string[])  [unwired: 4 in]
                        n2243 = call "Insert_empty_element_with_zero.vi"("searched date"=w12305, "fixed date"=w12303) -> ("O/P"=w12298:string[])  [unwired: 9 in]
                        n2244 = call "Insert_empty_element_with_zero.vi"("searched date"=w12301, "fixed date"=w12303) -> ("O/P"=w12304:string[])  [unwired: 9 in]
                      }
                      frame #2 {
                        n2245 = call "Stack_holderwise_total_bd_count_&_duration.vi"("Refnum in"=w12337, "BREAKDOWN_STK_HOLD_ID"=2, "condition"=w12327, "Form Date"=w12335, "To Date"=w12334, "error in (no error)"=w12339) -> ("Refnum out"=w12336:T2, "Count out"=w12333:string[], "appended array"=w12329:dbl[], "error out"=w12338:errorcluster)  [unwired: 6 in]
                        n2246 = call "Insert_empty_element_with_zero.vi"("searched date"=w12333, "fixed date"=w12330) -> ("O/P"=w12332:string[])  [unwired: 9 in]
                        n2247 = call "NUMERIC TO STRING.vi"("appended array"=w12329) -> ("Array"=w12328:string[])  [unwired: 4 in]
                        n2248 = call "Insert_empty_element_with_zero.vi"("searched date"=w12328, "fixed date"=w12330) -> ("O/P"=w12331:string[])  [unwired: 9 in]
                      }
                      frame #3 {
                        n2249 = disable-structure shown="Enabled" {
                          disable-tunnel: w12356 -> [w12370 w12373]
                          disable-tunnel: [w12369 w12373] -> w12355
                          disable-tunnel: w12354 -> [w12368 w12372]
                          disable-tunnel: [w12367 w12372] -> w12353
                          disable-tunnel: w12352 -> [w12366 _]
                          disable-tunnel: w12351 -> [w12365 _]
                          disable-tunnel: [w12364 _] -> w12350
                          disable-tunnel: [w12363 _] -> w12346
                          disable-tunnel: w12344 -> [w12362 _]
                          frame Disabled {
                            n2250 = call "Stack_holderwise_total_bd_count_&_duration.vi"("Refnum in"=w12368, "BREAKDOWN_STK_HOLD_ID"=3, "condition"=w12362, "Form Date"=w12366, "To Date"=w12365, "error in (no error)"=w12370) -> ("Refnum out"=w12367:T2, "Count out"=w12364:string[], "appended array"=w12363:dbl[], "error out"=w12369:errorcluster)  [unwired: 6 in]
                          }
                          frame Enabled {
                          }
                        }
                        n2251 = call "Insert_empty_element_with_zero.vi"("searched date"=w12350, "fixed date"=w12347) -> ("O/P"=w12349:string[])  [unwired: 9 in]
                        n2252 = call "NUMERIC TO STRING.vi"("appended array"=w12346) -> ("Array"=w12345:string[])  [unwired: 4 in]
                        n2253 = call "Insert_empty_element_with_zero.vi"("searched date"=w12345, "fixed date"=w12347) -> ("O/P"=w12348:string[])  [unwired: 9 in]
                      }
                      frame #4 {
                        n2254 = disable-structure shown="Enabled" {
                          disable-tunnel: w12387 -> [w12403 w12406]
                          disable-tunnel: w12386 -> [w12402 w12405]
                          disable-tunnel: [w12401 w12405] -> w12385
                          disable-tunnel: [w12400 w12406] -> w12384
                          disable-tunnel: w12383 -> [w12399 _]
                          disable-tunnel: w12382 -> [w12398 _]
                          disable-tunnel: [w12397 _] -> w12381
                          disable-tunnel: [w12396 _] -> w12377
                          disable-tunnel: w12375 -> [w12395 _]
                          frame Disabled {
                            n2255 = call "Stack_holderwise_total_bd_count_&_duration.vi"("Refnum in"=w12402, "BREAKDOWN_STK_HOLD_ID"=4, "condition"=w12395, "Form Date"=w12399, "To Date"=w12398, "error in (no error)"=w12403) -> ("Refnum out"=w12401:T2, "Count out"=w12397:string[], "appended array"=w12396:dbl[], "error out"=w12400:errorcluster)  [unwired: 6 in]
                          }
                          frame Enabled {
                          }
                        }
                        n2256 = call "Insert_empty_element_with_zero.vi"("searched date"=w12381, "fixed date"=w12378) -> ("O/P"=w12380:string[])  [unwired: 9 in]
                        n2257 = call "NUMERIC TO STRING.vi"("appended array"=w12377) -> ("Array"=w12376:string[])  [unwired: 4 in]
                        n2258 = call "Insert_empty_element_with_zero.vi"("searched date"=w12376, "fixed date"=w12378) -> ("O/P"=w12379:string[])  [unwired: 9 in]
                      }
                      frame #5 {
                        n2259 = disable-structure shown="Enabled" {
                          disable-tunnel: w12420 -> [w12438 w12441]
                          disable-tunnel: [w12437 w12441] -> w12419
                          disable-tunnel: w12418 -> [w12436 w12440]
                          disable-tunnel: [w12435 w12440] -> w12417
                          disable-tunnel: w12416 -> [w12434 _]
                          disable-tunnel: w12415 -> [w12433 _]
                          disable-tunnel: [w12432 _] -> w12414
                          disable-tunnel: [w12431 _] -> w12410
                          disable-tunnel: w12408 -> [w12430 _]
                          frame Disabled {
                            n2260 = call "Stack_holderwise_total_bd_count_&_duration.vi"("Refnum in"=w12436, "BREAKDOWN_STK_HOLD_ID"=5, "condition"=w12430, "Form Date"=w12433, "To Date"=w12434, "error in (no error)"=w12438) -> ("Refnum out"=w12435:T2, "Count out"=w12432:string[], "appended array"=w12431:dbl[], "error out"=w12437:errorcluster)  [unwired: 6 in]
                          }
                          frame Enabled {
                          }
                        }
                        n2261 = call "NUMERIC TO STRING.vi"("appended array"=w12410) -> ("Array"=w12409:string[])  [unwired: 4 in]
                        n2262 = call "Insert_empty_element_with_zero.vi"("searched date"=w12414, "fixed date"=w12412) -> ("O/P"=w12413:string[])  [unwired: 9 in]
                        n2263 = call "Insert_empty_element_with_zero.vi"("searched date"=w12409, "fixed date"=w12412) -> ("O/P"=w12411:string[])  [unwired: 9 in]
                      }
                      frame #6 {
                        n2264 = call "String to numeric.vi"("Array"=w12452) -> ("Array 2"=w12451:dbl[])  [unwired: 4 in]
                        n2265 = call "String to numeric.vi"("Array"=w12450) -> ("Array 2"=w12449:dbl[])  [unwired: 4 in]
                        n2266 = call "String to numeric.vi"("Array"=w12448) -> ("Array 2"=w12447:dbl[])  [unwired: 4 in]
                        n2267 = call "String to numeric.vi"("Array"=w12446) -> ("Array 2"=w12445:dbl[])  [unwired: 4 in]
                        n2268 = call "String to numeric.vi"("Array"=w12444) -> ("Array 2"=w12443:dbl[])  [unwired: 4 in]
                        n2269 = Decimal String To Number(string=w12457) -> (number=w12476:i32[])  [unwired: 2 in, 1 out]
                        n2270 = Decimal String To Number(string=w12458) -> (number=w12477:i32[])  [unwired: 2 in, 1 out]
                        n2271 = Decimal String To Number(string=w12459) -> (number=w12478:i32[])  [unwired: 2 in, 1 out]
                        n2272 = Decimal String To Number(string=w12460) -> (number=w12479:i32[])  [unwired: 2 in, 1 out]
                        n2273 = Decimal String To Number(string=w12461) -> (number=w12474:i32[])  [unwired: 2 in, 1 out]
                        n2274 = Compound Arithmetic op=ADD(w12451, w12449, w12447, w12445, w12443) -> (w12454:dbl[])
                        n2275 = Build Array(w12452) -> (w12473:string[][])
                        n2276 = Build Array(w12450) -> (w12472:string[][])
                        n2277 = Build Array(w12448) -> (w12471:string[][])
                        n2278 = Build Array(w12446) -> (w12470:string[][])
                        n2279 = Build Array(w12444) -> (w12469:string[][])
                        n2280 = Number To Fractional String(number=w12454, precision (6)=i16 2) -> (F-format string=w12453:string[])  [unwired: 2 in]
                        n2281 = Compound Arithmetic op=ADD(w12476, w12477, w12478, w12479, w12474) -> (w12480:i32[])
                        n2282 = Transpose 2D Array(2D array=w12473) -> (transposed array=w12467:string[][])
                        n2283 = Transpose 2D Array(2D array=w12472) -> (transposed array=w12466:string[][])
                        n2284 = Transpose 2D Array(2D array=w12471) -> (transposed array=w12465:string[][])
                        n2285 = Transpose 2D Array(2D array=w12470) -> (transposed array=w12464:string[][])
                        n2286 = Transpose 2D Array(2D array=w12469) -> (transposed array=w12463:string[][])
                        n2287 = Number To Decimal String(number=w12480) -> (decimal integer string=w12475:string[])  [unwired: 1 in]
                        n2288 = Build Array(w12453) -> (w12456:string[][])
                        n2289 = Transpose 2D Array(2D array=w12456) -> (transposed array=w12462:string[][])
                      }
                      frame #7 {
                        w12483 = string[] ["0"]
                        n2290 = Insert Into Array(array=w12493, index (col)=1 ("disabled index (col)"), new element #1=w12483, new element #2=w12483, new element #3=w12485, new element #4=w12484, new element #5=w12483, new element #6=w12483, new element #7=w12483, new element #8=w12483, new element #9=w12483, new element #10=w12483, new element #11=w12486, new element #12=w12487) -> (w12489:string[][])  [unwired: 1 in]
                        n2291 = call "flot graph for month n year.vi"("BD Date"=w12490, "error in (no error)"=w12492, "Count total"=w12486) -> ("error out"=w12491:errorcluster, "Run-Time Status"=w12488:cluster{"Array 2":timestamp[], dbl[]})  [unwired: 7 in]
                        n2292 = local write "Run-Time Status"(w12488) -> ()
                        n2293 = local write "Table"(w12489) -> ()
                      }
                    }
                  }
                  frame "1" {
                    n2294 = flat-sequence {
                      tunnel: w12505 -> [w12619]
                      tunnel: w12504 -> [w12617]
                      tunnel: [w12603] -> w12595
                      tunnel: [w12618] -> w12594
                      tunnel: w12503 -> [_]
                      tunnel: [w12622] -> w12593
                      tunnel: [w12602] -> w12592
                      tunnel: [w12601] -> w12591
                      tunnel: [w12600] -> w12590
                      tunnel: w12502 -> [w12602]
                      tunnel: w12501 -> [w12601]
                      tunnel: ["Where BREAKDOWN_DATE between '%s'and '%s' and BREAKDOWN_STK_HOLD_ID ='%d' and  SHIFT_ID = '%d' "] -> w12589
                      tunnel: [w12600] -> w12588
                      tunnel: w12500 -> [w12596]
                      tunnel: [w12596] -> w12499
                      tunnel: w12595 -> [w12683]
                      tunnel: w12594 -> [w12685]
                      tunnel: w12593 -> [w12681]
                      tunnel: w12592 -> [w12680]
                      tunnel: w12591 -> [w12679]
                      tunnel: [w12682] -> w12587
                      tunnel: [w12684] -> w12586
                      tunnel: [w12681] -> w12585
                      tunnel: [w12671] -> w12584
                      tunnel: [w12677] -> w12583
                      tunnel: [w12680] -> w12582
                      tunnel: [w12679] -> w12581
                      tunnel: w12590 -> [w12676]
                      tunnel: [w12676] -> w12580
                      tunnel: w12589 -> [w12673]
                      tunnel: [w12673] -> w12579
                      tunnel: [w12672] -> w12578
                      tunnel: w12588 -> [w12672]
                      tunnel: w12499 -> [w12670]
                      tunnel: [w12669] -> w12498
                      tunnel: w12587 -> [w12715]
                      tunnel: w12586 -> [w12713]
                      tunnel: w12585 -> [w12718]
                      tunnel: w12584 -> [w12717]
                      tunnel: w12583 -> [w12716]
                      tunnel: w12582 -> [w12711]
                      tunnel: w12581 -> [w12710]
                      tunnel: [w12718] -> w12577
                      tunnel: [w12717] -> w12576
                      tunnel: [w12716] -> w12575
                      tunnel: [w12714] -> w12574
                      tunnel: [w12708] -> w12573
                      tunnel: [w12707] -> w12572
                      tunnel: [w12712] -> w12571
                      tunnel: [w12711] -> w12570
                      tunnel: [w12710] -> w12569
                      tunnel: w12580 -> [w12706]
                      tunnel: [w12706] -> w12568
                      tunnel: w12579 -> [w12703]
                      tunnel: [w12703] -> w12567
                      tunnel: [w12702] -> w12566
                      tunnel: w12578 -> [w12702]
                      tunnel: w12498 -> [w12700]
                      tunnel: w12577 -> [w12737]
                      tunnel: w12576 -> [w12736]
                      tunnel: w12575 -> [w12735]
                      tunnel: w12574 -> [w12732]
                      tunnel: w12573 -> [w12734]
                      tunnel: w12572 -> [w12733]
                      tunnel: w12571 -> [w12730]
                      tunnel: w12570 -> [w12728]
                      tunnel: w12569 -> [w12727]
                      tunnel: [w12737] -> w12565
                      tunnel: [w12736] -> w12564
                      tunnel: [w12735] -> w12563
                      tunnel: [w12734] -> w12562
                      tunnel: [w12733] -> w12561
                      tunnel: [w12731] -> w12560
                      tunnel: [w12725] -> w12559
                      tunnel: [w12724] -> w12558
                      tunnel: [w12729] -> w12557
                      tunnel: [w12728] -> w12556
                      tunnel: [w12727] -> w12555
                      tunnel: w12568 -> [w12723]
                      tunnel: [w12723] -> w12554
                      tunnel: w12567 -> [w12720]
                      tunnel: [w12720] -> w12553
                      tunnel: [w12719] -> w12552
                      tunnel: w12566 -> [w12719]
                      tunnel: w12565 -> [w12770]
                      tunnel: w12564 -> [w12769]
                      tunnel: w12563 -> [w12768]
                      tunnel: w12562 -> [w12767]
                      tunnel: w12561 -> [w12766]
                      tunnel: w12560 -> [w12763]
                      tunnel: w12559 -> [w12765]
                      tunnel: w12558 -> [w12764]
                      tunnel: w12557 -> [w12762]
                      tunnel: w12556 -> [w12759]
                      tunnel: w12555 -> [w12758]
                      tunnel: [w12770] -> w12551
                      tunnel: [w12769] -> w12550
                      tunnel: [w12768] -> w12549
                      tunnel: [w12767] -> w12548
                      tunnel: [w12766] -> w12547
                      tunnel: [w12765] -> w12546
                      tunnel: [w12764] -> w12545
                      tunnel: [w12761] -> w12544
                      tunnel: [w12760] -> w12543
                      tunnel: [w12756] -> w12542
                      tunnel: [w12755] -> w12541
                      tunnel: [w12759] -> w12540
                      tunnel: [w12758] -> w12539
                      tunnel: w12554 -> [w12754]
                      tunnel: [w12754] -> w12538
                      tunnel: w12553 -> [w12751]
                      tunnel: [w12751] -> w12537
                      tunnel: [w12750] -> w12536
                      tunnel: w12552 -> [w12750]
                      tunnel: w12551 -> [w12805]
                      tunnel: w12550 -> [w12804]
                      tunnel: w12549 -> [w12803]
                      tunnel: w12548 -> [w12802]
                      tunnel: w12547 -> [w12801]
                      tunnel: w12546 -> [w12800]
                      tunnel: w12545 -> [w12799]
                      tunnel: w12544 -> [w12794]
                      tunnel: w12543 -> [w12796]
                      tunnel: w12542 -> [w12798]
                      tunnel: w12541 -> [w12797]
                      tunnel: w12540 -> [w12791]
                      tunnel: w12539 -> [w12792]
                      tunnel: [w12805] -> w12535
                      tunnel: [w12804] -> w12534
                      tunnel: [w12803] -> w12533
                      tunnel: [w12802] -> w12532
                      tunnel: [w12801] -> w12531
                      tunnel: [w12800] -> w12530
                      tunnel: [w12799] -> w12529
                      tunnel: [w12798] -> w12528
                      tunnel: [w12797] -> w12527
